vi "Functional Imaging-Add Z-stack images handler.vi"(8 "error in (no error)":errorcluster) -> (0 "error out":errorcluster)   [LabVIEW 2013]
uses:
  Typedefs/Overlay FG functions.ctl
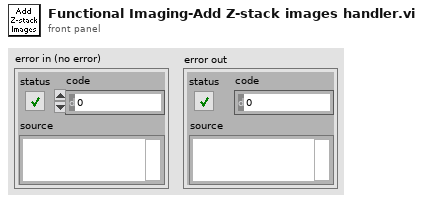
[diagram p1: front panel]
types:
  T1 = typedef "Overlay FG functions.ctl" = enum16{"Generate new images", "Get stored images", "Clear"}
  T2 = typedef "IMAQ Image.ctl" = refnum<image>
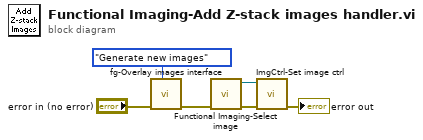
[diagram p0: block diagram]
diagram:
  n1 = call "fg-Overlay images interface.vi"("Function"=Overlay_FG_functions."Generate new images", "error in (no error)"="error in (no error)") -> ("error out"=w6:errorcluster)  [unwired: 7 in, 2 out]
  n2 = call "Functional Imaging-Select image.vi"("error in (no error)"=w6) -> ("error out"=w3:errorcluster, "SelectedPOIMax"=w1:T2)  [unwired: 9 in]
  n3 = call "ImgCtrl-Set image ctrl.vi"("error in"=w3, "Image"=w1) -> ("error out"=→"error out":errorcluster)  [unwired: 9 in]
